vi "Create Error Log Text.vi"(2 "Error_Log_Setting":T1, 3 "Error to be logged":T2) -> (0 "Number of characters":i32, 1 "Text to be written to error log file":string)   [LabVIEW 2023, in "Error Manager.lvlib" / "Error Log.lvclass"]
uses:
  Error Log.lvclass
  Error to be logged (cluster).ctl
  Error Type (enum).ctl
  Error Log.lvclass/Error Log.ctl
  Settings/Error_Log_Setting (enum).ctl
  Settings/Settings.lvclass
panel:
  # "Input\nInputs to the VI"
  # "Development\nControls or indicators that are useful for development or testing, but which are not outputs of the VI."
  # "Output\nOutputs of the VI"
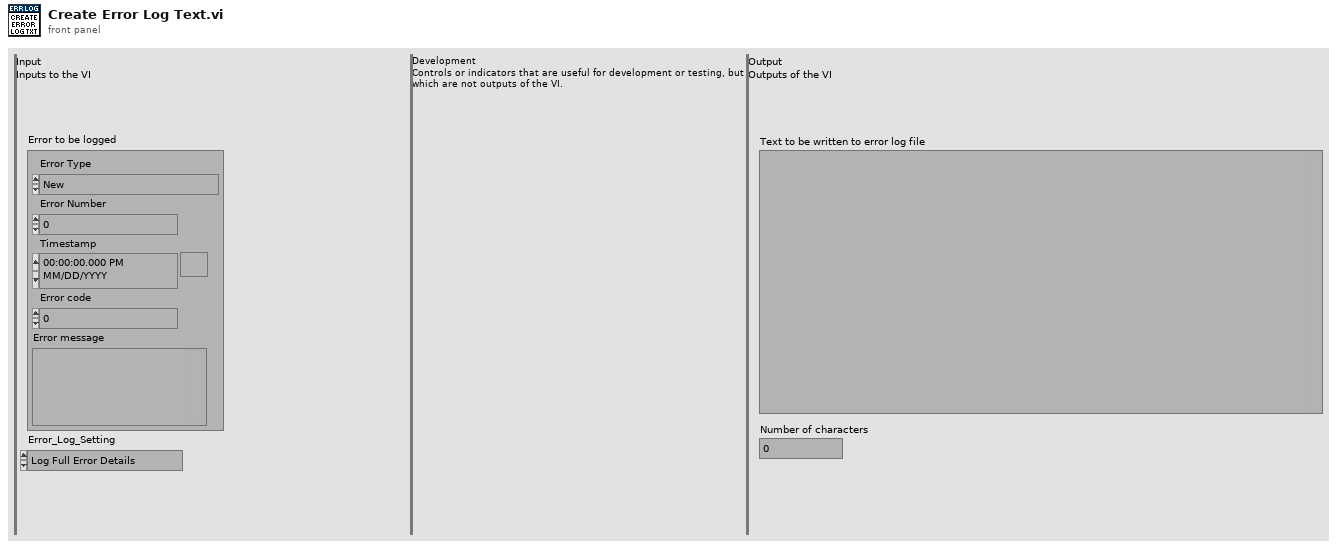
[diagram p1: front panel]
types:
  T1 = typedef "Error Manager.lvlib/Settings.lvclass/Error_Log_Setting (enum).ctl" = enum16{"Log Full Error Details", "Log Error Codes Only", "Do Not Log"}
  T2 = typedef "Error Manager.lvlib/Error Log.lvclass/Error to be logged (cluster).ctl" = cluster{"Error Type":T3, "Error Number":i32, "Timestamp":timestamp, "Error code":i32, "Error message":string}
  T3 = typedef "Error Manager.lvlib/Error Log.lvclass/Error Type (enum).ctl" = enum16{"New", "Identical to last logged error"}
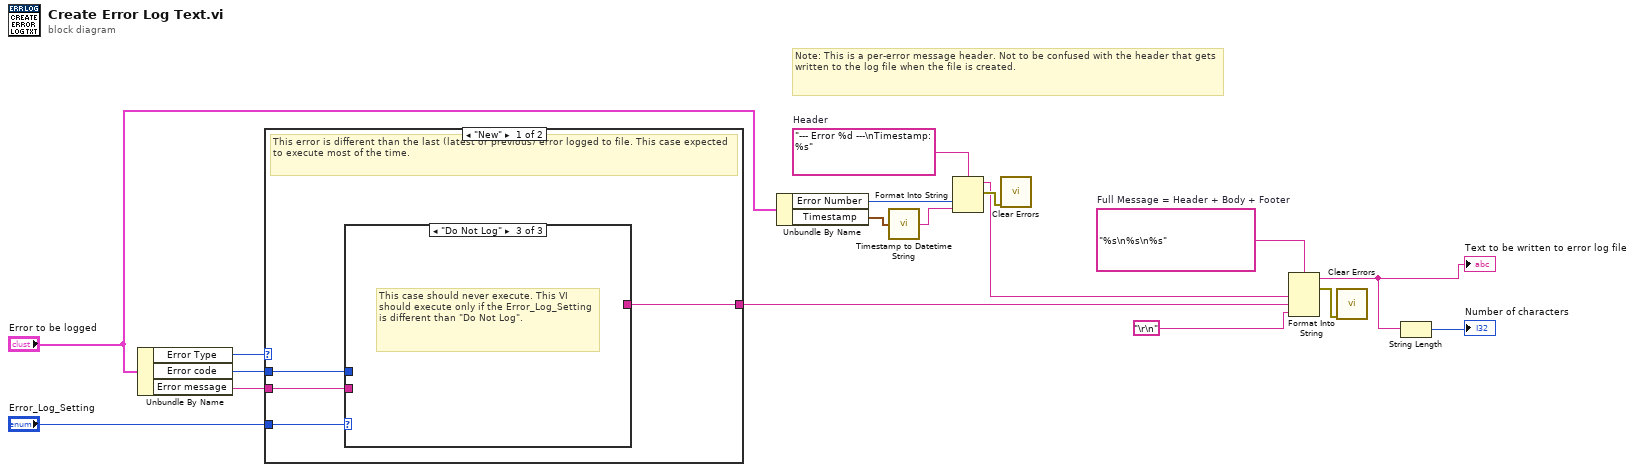
[diagram p0: block diagram]
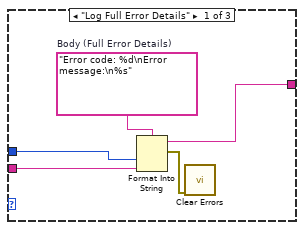
[diagram p2: hidden frame]
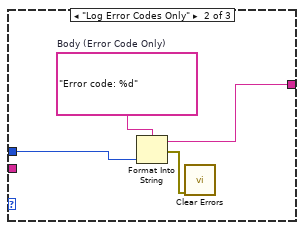
[diagram p3: hidden frame]
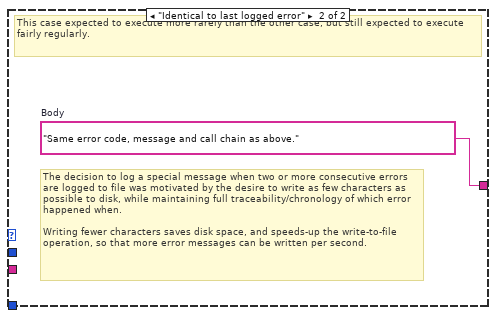
[diagram p4: hidden frame]
diagram:
  w8 = "%s\n%s\n%s"  # Full Message = Header + Body + Footer
  w14 = "--- Error %d ---\nTimestamp: %s"  # Header
  # "Note: This is a per-error message header. Not to be confused with the header that gets written to the log file when the file is created."
  n1 = Unbundle By Name("Error to be logged") -> ("Error Type"=w15:T3, "Error code"=w17:i32, "Error message"=w16:string)
  n2 = case shown="\"New\"" w15 {
    tunnel: [w21 w31] -> w6
    tunnel: w17 -> [w20 _]
    tunnel: w16 -> [w19 _]
    tunnel: "Error_Log_Setting" -> [w18 _]
    frame "New" {
      # "This error is different than the last (latest or previous) error logged to file. This case expected to execute most of the time."
      n3 = case shown="\"Do Not Log\"" w18 {
        tunnel: [w25 w29 _] -> w21
        tunnel: w20 -> [w23 w27 _]
        tunnel: w19 -> [w22 _ _]
        frame "Log Full Error Details" {
          w26 = "Error code: %d\nError message:\n%s"  # Body (Full Error Details)
          n4 = Format Into String(format string=w26, w23, w22) -> (resulting string=w25:string, error out=w24:errorcluster)  [unwired: 2 in]
          n5 = call <vilib>:"Clear Errors.vi"("error in (no error)"=w24) -> ()  [unwired: 5 in, 2 out]
        }
        frame "Log Error Codes Only" {
          w30 = "Error code: %d"  # Body (Error Code Only)
          n6 = Format Into String(format string=w30, w27) -> (resulting string=w29:string, error out=w28:errorcluster)  [unwired: 2 in]
          n7 = call <vilib>:"Clear Errors.vi"("error in (no error)"=w28) -> ()  [unwired: 5 in, 2 out]
        }
        frame "Do Not Log" {
          # "This case should never execute. This VI should execute only if the Error_Log_Setting is different than \"Do Not Log\"."
        }
      }
    }
    frame "Identical to last logged error" {
      w31 = "Same error code, message and call chain as above."  # Body
      # "The decision to log a special message when two or more consecutive errors are logged to file was motivated by the desire to write as few characters as possible to disk, while maintaining full traceability/chronology of which error happened when.\n\nWriting fewer characters saves disk space, and speeds-up the write-to-file operation, so that more error messages can be written per second."
      # "This case expected to execute more rarely than the other case, but still expected to execute fairly regularly."
    }
  }
  n8 = Unbundle By Name("Error to be logged") -> ("Error Number"=w12:i32, "Timestamp"=w11:timestamp)
  n9 = call "Timestamp to Datetime String.vi"("Timestamp"=w11) -> ("Date-Time String"=w10:string)
  n10 = Format Into String(format string=w14, w12, w10) -> (resulting string=w7:string, error out=w9:errorcluster)  [unwired: 2 in]
  n11 = call <vilib>:"Clear Errors.vi"("error in (no error)"=w9) -> ()  [unwired: 5 in, 2 out]
  n12 = Format Into String(format string=w8, w7, w6, "\r\n") -> (resulting string=w3:string, error out=w4:errorcluster)  [unwired: 2 in]
  "Text to be written to error log file" <- w3
  n13 = call <vilib>:"Clear Errors.vi"("error in (no error)"=w4) -> ()  [unwired: 5 in, 2 out]
  n14 = String Length(string=w3) -> (length=→"Number of characters":i32)
